vi "TTT_AI.vi"() -> ()   [LabVIEW 2017]
panel:
  in  "Registerkarte":enum32{"Start", "Begr", "spiel", "info"}(tab)
  in  "Eingabe":bool
  in  "Name":string
  out "AnzeigeBegrüß":string
  in  "Registerkarte 2":enum32{"Seite 1"}(tab)
  in  "Panel Farbe":u32(colorbox)
  in  "Panel Farbe 2":u32
  in  "Boolesch":bool
  in  "info1":bool
  in  "spieler1":bool
  out "Ring":u16(ring)
  out "Scoreboard":T1(tab)
  out "Leicht":T2
  out "Mittel":T3
  out "Unmöglich":T3
  out "Mit Fruende":T3
  out "Ausgabe":string
  out "Scoring":bool
  out "O Zug":bool
  in  "X Zug":bool
  in  "BoolArray":bool[][](array[boolean])
  out "Array":i8[][](array[ring])
  in  "Zeile x Spalte":i8=3 min=3 max=3
  in  "stop":bool
  in  "NSpiel":bool
  out "ShowLed":bool
  out "SBeendet":bool
  out "NZueg":i8
  out "O Gewonen":bool
  out "X Gewonen":bool
  in  "Enum":T4(ring)
  in  "zurück":bool
  out "String":string
  out "hidenArray":u8[][](array[numeric])
  # "Geben Sie Ihre Name ein"
  # "Nächte Zug"
  # "Farbe Ändern"
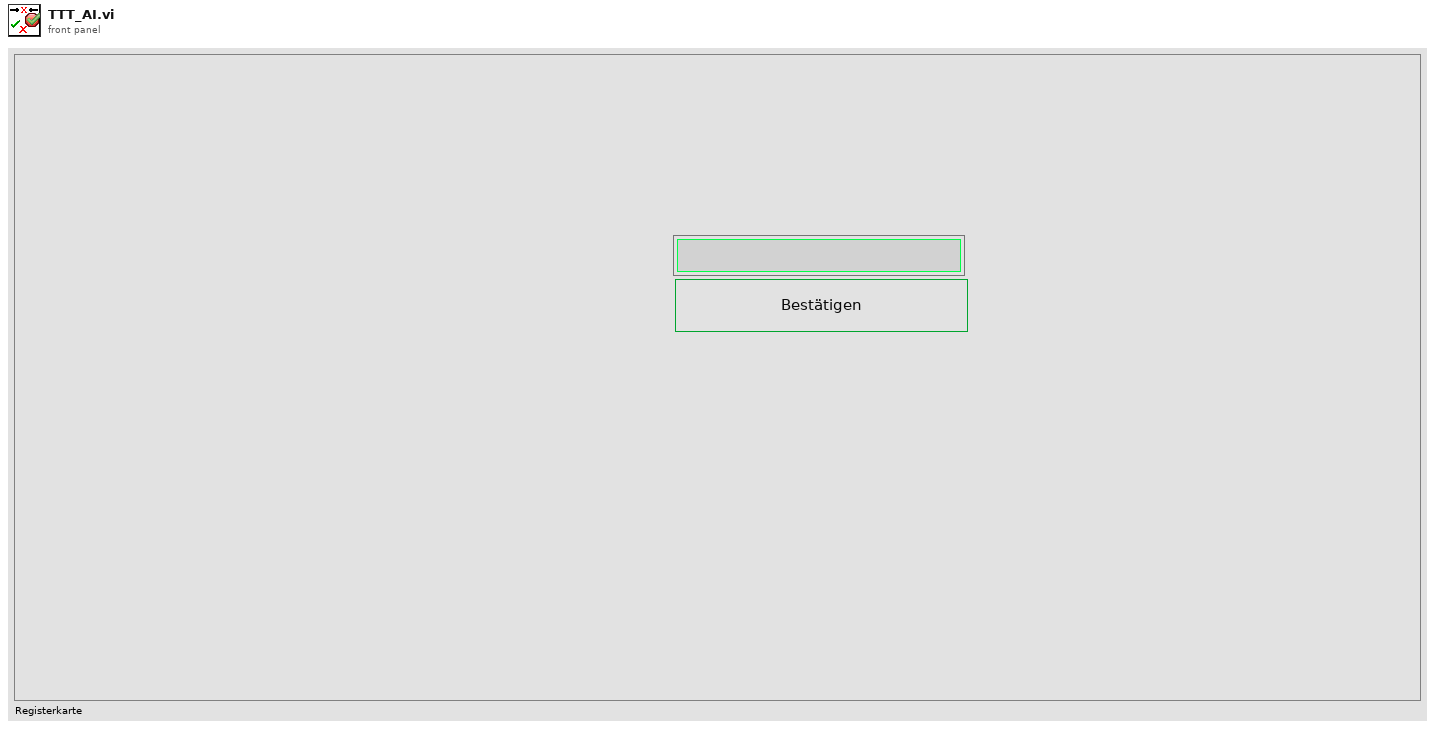
[diagram p1: front panel]
types:
  T1 = enum32{"Seite 1", "Seite 2", "Seite 3", "Seite 4"}
  T2 = cluster{"Spieler":u32, "Gegner":u32, "Unenschieden":u32}
  T3 = cluster{"Spieler":u32, "System":u32, "Unenschieden":u32}
  T4 = enum16{"Leicht", "Mittel", "Unmöglich", "Mit einem Freund Spielen"}
  T5 = enum8{"Enabled", "Disabled", "Disabled and Grayed Out"}
  T6 = cluster{"Spieler":dbl, "Rechner":dbl, "Draw":dbl}
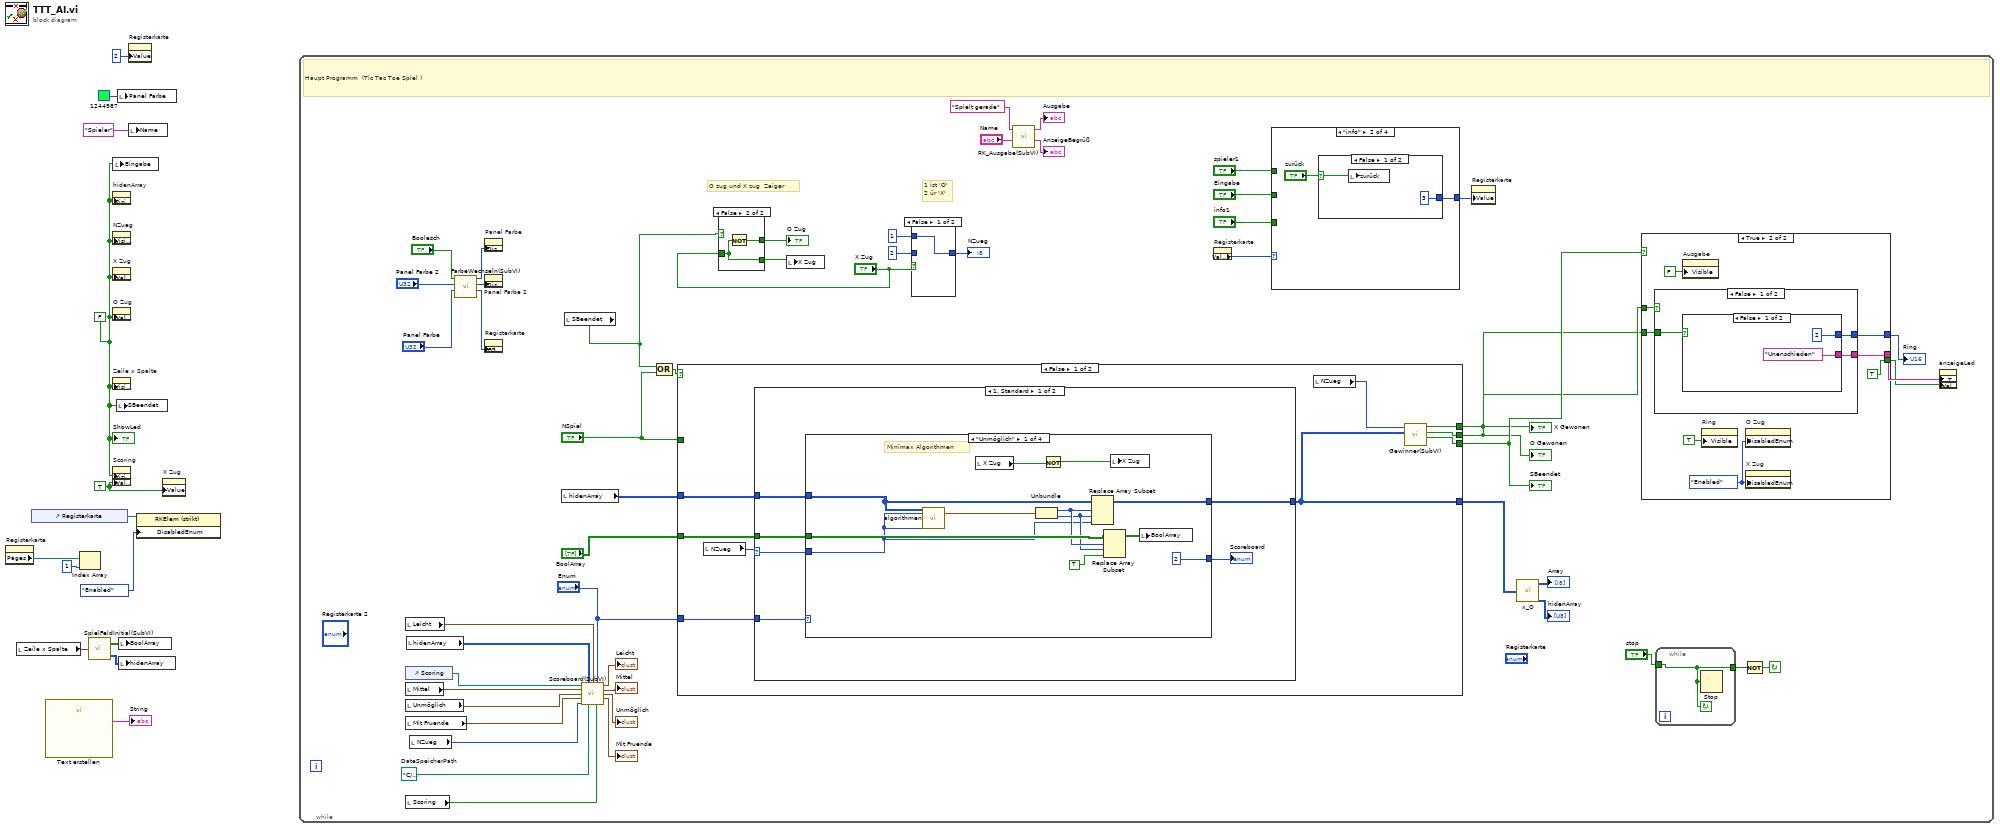
[diagram p0: block diagram]
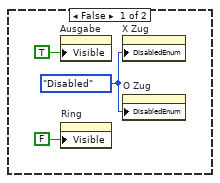
[diagram p3: hidden frame]
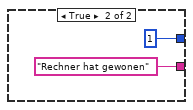
[diagram p4: hidden frame]
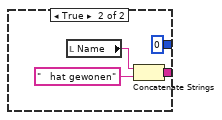
[diagram p5: hidden frame]
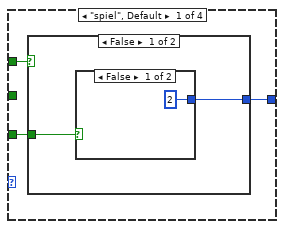
[diagram p6: hidden frame]
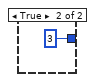
[diagram p7: hidden frame]
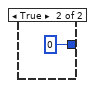
[diagram p8: hidden frame]
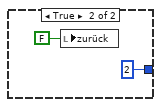
[diagram p9: hidden frame]
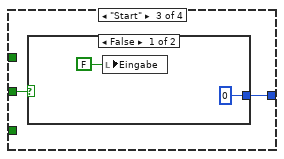
[diagram p10: hidden frame]
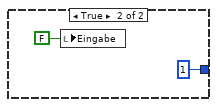
[diagram p11: hidden frame]
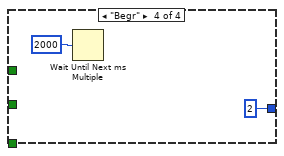
[diagram p12: hidden frame]
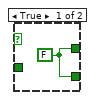
[diagram p13: hidden frame]
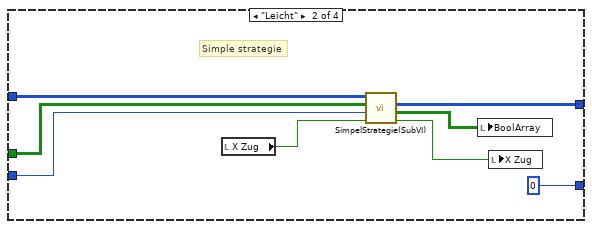
[diagram p14: hidden frame]
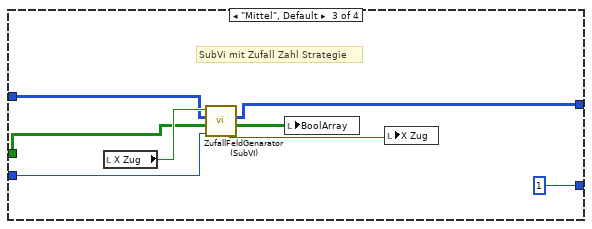
[diagram p15: hidden frame]
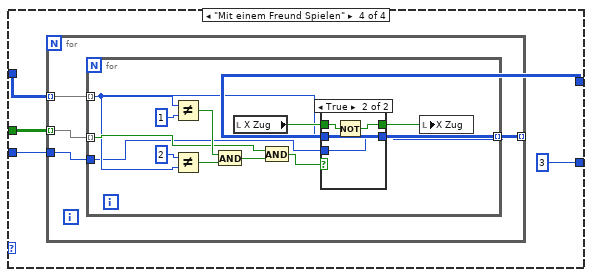
[diagram p16: hidden frame]
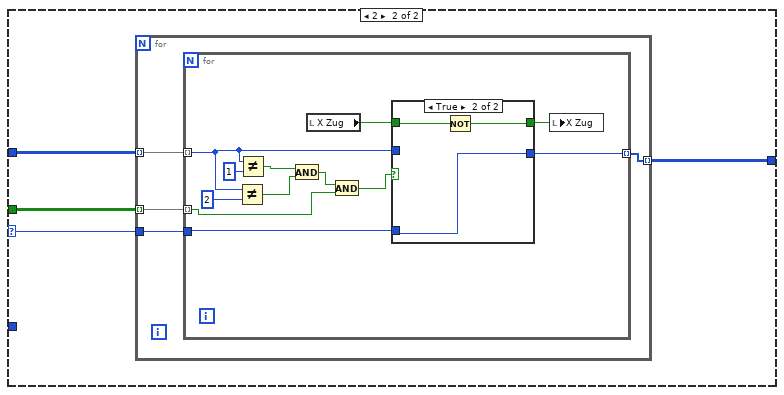
[diagram p18: hidden frame]
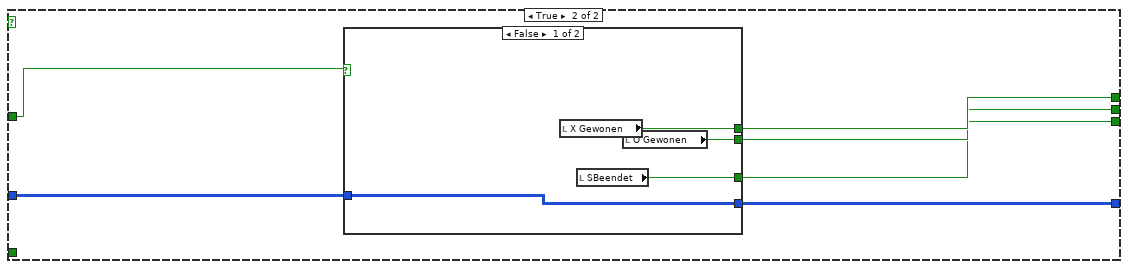
[diagram p20: hidden frame]
diagram:
  w2 = FALSE
  w1 = TRUE
  n1 = property on="Registerkarte" class="RKElem (strikt)"() -> ("Pages"=w6:refnum<vi>[])  [unwired: 2 in, 2 out]
  n2 = local read "Zeile x Spalte"() -> (w13:i8)
  n3 = control-ref of="Registerkarte"() -> (w5:refnum<vi>)
  n4 = call "Text erstellen"() -> ("Result"=→"String":string)  [unwired: 14 in, 1 out]
  n5 = Index Array(array=w6, index=1 ("Index")) -> ()  [unwired: 1 out]
  n6 = call "SpielFeldInitial(SubVI).vi"("SpalteUndZeile"=w13) -> ("TictactoeFelder"=w12:bool[][], "Grafikring"=w11:i8[][])
  n7 = local write "Eingabe"(w2) -> ()
  n8 = property on="hidenArray" class="Arr (strikt)"("Visible"=w2) -> ()  [unwired: 2 in, 2 out]
  n9 = property on="NZueg" class="DigWert (strikt)"("Visible"=w2) -> ()  [unwired: 2 in, 2 out]
  n10 = property on="X Zug" class="Bool. (strikt)"("Value"=w2) -> ()  [unwired: 2 in, 2 out]
  n11 = property on="O Zug" class="Bool. (strikt)"("Value"=w2) -> ()  [unwired: 2 in, 2 out]
  n12 = property on="Zeile x Spalte" class="DigWert (strikt)"("Visible"=w2) -> ()  [unwired: 2 in, 2 out]
  n13 = property on="Scoring" class="Bool. (strikt)"("Visible"=w2, "Value"=w1) -> ()  [unwired: 2 in, 2 out]
  n14 = local write "SBeendet"(w2) -> ()
  n15 = local write "Panel Farbe"(u32 1244987 ("Panel Farbe")) -> ()
  n16 = local write "BoolArray"(w12) -> ()
  n17 = local write "hidenArray"(w11) -> ()
  n18 = property on="Registerkarte" class="RKElem (strikt)"("Value"=2) -> ()  [unwired: 2 in, 2 out]
  n19 = local write "Name"("Spieler") -> ()
  n20 = property class="RKElem (strikt)"(reference=w5, "DisabledEnum"=T5."Enabled" ("Deaktiviert")) -> ()  [unwired: 1 in, 2 out]
  n21 = property on="X Zug" class="Bool. (strikt)"("Value"=w1) -> ()  [unwired: 2 in, 2 out]
  n22 = while {
    stop <- w57 continue-if-true
    w35 = path "C:/Users/MohammadZahirul/Desktop/TicTacToe_Doc/projekt_tictactoe/Ergebnis.txt"  # DateSpeicherPath
    # "O zug und X zug  Zeiger"
    # "1 ist 'O'\n2 ür 'X'"
    # "Haupt Programm  (Tic Tac Toe Spiel )"
    n23 = local read "Leicht"() -> (w55:T2)
    n24 = control-ref of="Scoring"() -> (w43:refnum<vi>)
    n25 = local read "Mittel"() -> (w54:T3)
    n26 = local read "Unmöglich"() -> (w53:T3)
    n27 = local read "Mit Fruende"() -> (w52:T3)
    n28 = local read "Scoring"() -> (w56:bool)
    n29 = local read "hidenArray"() -> (w33:u8[][])
    n30 = local read "NZueg"() -> (w36:i8)
    n31 = call "FarbeWechseln(SubVI).vi"("Panel Farbe"="Panel Farbe", "Panel Farbe 2"="Panel Farbe 2", "Boolesch"="Boolesch") -> ("Panel Farbe 3"=w39:u32, "Deaktiviert 2"=w42:T5, "Deaktiviert"=w40:T5)  [unwired: 6 in]
    n32 = property on="Panel Farbe" class="Farbfeld"("DisabledEnum"=w40) -> ()  [unwired: 2 in, 2 out]
    n33 = property on="Panel Farbe 2" class="DigWert (strikt)"("DisabledEnum"=w42) -> ()  [unwired: 2 in, 2 out]
    n34 = property on="Registerkarte" class="RKElem (strikt)"("FG Color"=w39) -> ()  [unwired: 2 in, 2 out]
    n35 = local read "hidenArray"() -> (w34:u8[][])
    n36 = local read "SBeendet"() -> (w20:bool)
    n37 = call "Scoreboard(SubVI).vi"("Boolean (Eingang)"=w43, "Tic Tac Toe (Eingang)"=w33, "Leicht"=w55, "Enum"="Enum", "Mittel"=w54, "Unmöglich"=w53, "Mit Fruende"=w52, "Next Turn"=w36, "DateSpeicherPath"=w35, "Ergebnis"=w56) -> ("Score 5"=→"Leicht":T6, "Score 6"=→"Mittel":T6, "Score 7"=→"Unmöglich":T6, "Score 8"=→"Mit Fruende":T6)  [unwired: 2 in]
    n38 = Compound Arithmetic op=OR ("Mehrfacharithmetik")(w20, "NSpiel") -> (w65:bool)
    n39 = case shown="False" w65 {
      tunnel: [w122 w215] -> w30
      tunnel: "BoolArray" -> [w124 _]
      tunnel: [w123 w214] -> w29
      tunnel: "NSpiel" -> [_ w211]
      tunnel: w34 -> [w121 w212]
      tunnel: [w119 w213] -> w61
      tunnel: [w120 w210] -> w31
      tunnel: "Enum" -> [w116 _]
      frame False {
        n40 = local read "NZueg"() -> (w117:i8)
        n41 = case shown="1, Standard" w117 {
          selector: w117 -> [w129 w186]
          tunnel: w124 -> [w130 w187]
          tunnel: w121 -> [w128 w188]
          tunnel: [w127 w185] -> w119
          tunnel: w116 -> [w125 _]
          frame 1, Default {
            n42 = case shown="\"Unmöglich\"" w125 {
              tunnel: w130 -> [w140 w146 w156 w163]
              tunnel: w129 -> [w137 w145 w152 w162]
              tunnel: w128 -> [w141 w147 w154 w161]
              tunnel: [w135 w150 w153 w160] -> w127
              tunnel: [2 0 1 3] -> w126
              frame "Unmöglich" {
                # "Minimax Algorithmen"
                n43 = call "algorithmen.vi"("Game"=w141, "Active Turn"=w137, "NextTurn"=w137) -> ("Next Move"=w142:cluster{"Row":i32, "Col":i32})  [unwired: 13 in, 3 out]
                n44 = local read "X Zug"() -> (w133:bool)
                n45 = Unbundle(w142) -> ("Row"=w139:i32, "Col"=w138:i32)
                n46 = Not(x=w133) -> (.not. x?=w132:bool)
                n47 = Replace Array Subset(array=w141, new element=w137, index (row)=w139, index (col)=w138) -> (w135:u8[][])
                n48 = Replace Array Subset(array=w140, new element=TRUE, index (row)=w139, index (col)=w138) -> (w134:bool[][])
                n49 = local write "X Zug"(w132) -> ()
                n50 = local write "BoolArray"(w134) -> ()
              }
              frame "Leicht" {
                # "Simple strategie"
                n51 = local read "X Zug"() -> (w144:bool)
                n52 = call "SimpelStrategie(SubVI).vi"("toggle"=w144, "NextTurn"=w145, "BoolArray"=w146, "Array"=w147) -> ("toggle 2"=w148:bool, "Array 3"=w149:bool[][], "Array 2"=w150:u8[][])  [unwired: 1 in]
                n53 = local write "BoolArray"(w149) -> ()
                n54 = local write "X Zug"(w148) -> ()
              }
              frame "Mittel", Default {
                # "SubVi mit Zufall Zahl Strategie"
                n55 = local read "X Zug"() -> (w157:bool)
                n56 = call "ZufallFeldGenarator (SubVI).vi"("Numerisch"=w152, "BoolArray (Eingang)"=w156, "Tic Tac Toe (Eingang)"=w154, "Toggle turn (Eingang)"=w157) -> ("BoolArray (Ausgang)"=w155:bool[][], "Tic Tac Toe (Ausgang)"=w153:u8[][], "Toggle turn (Ausgang)"=w158:bool)  [unwired: 1 in]
                n57 = local write "BoolArray"(w155) -> ()
                n58 = local write "X Zug"(w158) -> ()
              }
              frame "Mit einem Freund Spielen" {
                n59 = for {
                  tunnel: w163 -> [w167] mode=indexing
                  tunnel: w162 -> [w166]
                  tunnel: w161 -> [w165] mode=indexing
                  tunnel: [w164] -> w160 mode=indexing
                  n60 = for {
                    tunnel: w167 -> [w176] mode=indexing
                    tunnel: w166 -> [w168]
                    tunnel: w165 -> [w170] mode=indexing
                    tunnel: [w169] -> w164 mode=indexing
                    n61 = Not Equal?(x=w170, y=1) -> (x != y?=w179:bool)
                    n62 = Not Equal?(x=2, y=w170) -> (x != y?=w178:bool)
                    n63 = And(x=w179, y=w178) -> (x .and. y?=w177:bool)
                    n64 = local read "X Zug"() -> (w173:bool)
                    n65 = And(x=w176, y=w177) -> (x .and. y?=w175:bool)
                    n66 = case shown="True" w175 {
                      tunnel: [w181 w184] -> w174
                      tunnel: w173 -> [w181 w183]
                      tunnel: [w180 w182] -> w169
                      tunnel: w170 -> [w180 _]
                      tunnel: w168 -> [_ w182]
                      frame False {
                      }
                      frame True {
                        n67 = Not(x=w183) -> (.not. x?=w184:bool)
                      }
                    }
                    n68 = local write "X Zug"(w174) -> ()
                  }
                }
              }
            }
            "Scoreboard" <- w126
          }
          frame 2 {
            n69 = for {
              tunnel: w188 -> [w192] mode=indexing
              tunnel: w187 -> [w191] mode=indexing
              tunnel: w186 -> [w190]
              tunnel: [w189] -> w185 mode=indexing
              n70 = for {
                tunnel: w192 -> [w195] mode=indexing
                tunnel: w191 -> [w199] mode=indexing
                tunnel: w190 -> [w197]
                tunnel: [w196] -> w189 mode=indexing
                n71 = Not Equal?(x=w195, y=u8 2) -> (x != y?=w201:bool)
                n72 = Not Equal?(x=w195, y=u8 1) -> (x != y?=w202:bool)
                n73 = And(x=w202, y=w201) -> (x .and. y?=w200:bool)
                n74 = local read "X Zug"() -> (w194:bool)
                n75 = And(x=w200, y=w199) -> (x .and. y?=w198:bool)
                n76 = case shown="True" w198 {
                  tunnel: w197 -> [_ w209]
                  tunnel: [w206 w209] -> w196
                  tunnel: w195 -> [w206 _]
                  tunnel: w194 -> [w205 w207]
                  tunnel: [w205 w208] -> w193
                  frame False {
                  }
                  frame True {
                    n77 = Not(x=w207) -> (.not. x?=w208:bool)
                  }
                }
                n78 = local write "X Zug"(w193) -> ()
              }
            }
          }
        }
        n79 = local read "NZueg"() -> (w118:i8)
        n80 = call "Gewinner(SubVI).vi"("Array"=w119, "Next Turn"=w118) -> ("Game over"=w120:bool, "Win 2"=w123:bool, "Win"=w122:bool)  [unwired: 7 in]
      }
      frame True {
        n81 = case shown="False" w211 {
          tunnel: [w218 w226] -> w215
          tunnel: [w219 w226] -> w214
          tunnel: [w217 w223] -> w213
          tunnel: w212 -> [w217 _]
          tunnel: [w216 w226] -> w210
          frame False {
            n82 = local read "X Gewonen"() -> (w218:bool)
            n83 = local read "SBeendet"() -> (w216:bool)
            n84 = local read "O Gewonen"() -> (w219:bool)
          }
          frame True {
            w226 = FALSE
            n85 = property on="X Zug" class="Bool. (strikt)"("Value"=TRUE) -> ()  [unwired: 2 in, 2 out]
            n86 = call "SpielFeldInitial(SubVI).vi"("SpalteUndZeile"="Zeile x Spalte") -> ("TictactoeFelder"=w224:bool[][], "Grafikring"=w223:i8[][])
            n87 = local write "NZueg"(i8 2 ("Next Turn")) -> ()
            n88 = local write "BoolArray"(w224) -> ()
            "Scoring" <- TRUE
          }
        }
      }
    }
    "X Gewonen" <- w30
    "O Gewonen" <- w29
    "SBeendet" <- w31
    n89 = case shown="False" w20 {
      tunnel: [w112 w114] -> w22
      tunnel: [w112 w113] -> w23
      tunnel: "X Zug" -> [_ w114]
      frame True {
        w112 = FALSE
      }
      frame False {
        n90 = Not(x=w114) -> (.not. x?=w113:bool)
      }
    }
    "O Zug" <- w23
    n91 = local write "X Zug"(w22) -> ()
    n92 = case shown="False" "X Zug" {
      tunnel: [w66 w67] -> w26
      tunnel: 1 -> [w66 _]
      tunnel: 2 -> [_ w67]
      frame False {
      }
      frame True {
      }
    }
    "NZueg" <- w26
    n93 = call "RK_Ausgabe(SubVI).vi"("Name"="Name", "werS"="Spielt gerade") -> ("AnzeigeBegrüß"=→"AnzeigeBegrüß":string, "AnzeigeOben"=→"Ausgabe":string)  [unwired: 8 in]
    n94 = property on="Registerkarte" class="RKElem (strikt)"() -> ("Value"=w60:enum32{"Start", "Begr", "spiel", "info"})  [unwired: 2 in, 2 out]
    n95 = case shown="\"info\"" w60 {
      tunnel: [w92 w98 w105 2] -> w17
      tunnel: "Eingabe" -> [_ _ w104 _]
      tunnel: "spieler1" -> [w91 _ _ _]
      tunnel: "info1" -> [w90 _ _ _]
      frame "spiel", Default {
        n96 = case shown="False" w91 {
          tunnel: [w94 0] -> w92
          tunnel: w90 -> [w93 _]
          frame False {
            n97 = case shown="False" w93 {
              tunnel: [2 3] -> w94
              frame False {
              }
              frame True {
              }
            }
          }
          frame True {
          }
        }
      }
      frame "info" {
        n98 = case shown="False" "zurück" {
          selector: "zurück" -> [w100 _]
          tunnel: [3 2] -> w98
          frame False {
            n99 = local write "zurück"(w100) -> ()
          }
          frame True {
            n100 = local write "zurück"(FALSE) -> ()
          }
        }
      }
      frame "Start" {
        n101 = case shown="False" w104 {
          tunnel: [0 1] -> w105
          frame False {
            n102 = local write "Eingabe"(FALSE) -> ()
          }
          frame True {
            n103 = local write "Eingabe"(FALSE) -> ()
          }
        }
      }
      frame "Begr" {
        n104 = Wait Until Next ms Multiple(millisecond multiple=u32 2000 ("ms")) -> ()  [unwired: 1 out]
      }
    }
    n105 = property on="Registerkarte" class="RKElem (strikt)"("Value"=w17) -> ()  [unwired: 2 in, 2 out]
    n106 = call "x_O.vi"("Tic Tac Toe"=w61) -> ("GrafikRing"=→"Array":i32[][], "Game"=→"hidenArray":i32[][])  [unwired: 8 in]
    n107 = case shown="True" w31 {
      tunnel: w30 -> [_ w78]
      tunnel: w29 -> [_ w77]
      tunnel: [_ w76] -> w28
      tunnel: [_ w74] -> w27
      tunnel: [_ TRUE] -> w18
      frame False {
        w69 = T5."Disabled" ("Deaktiviert")
        n108 = property on="Ausgabe" class="Str"("Visible"=TRUE ("Sichtbar")) -> ()  [unwired: 2 in, 2 out]
        n109 = property on="Ring" class="Ring (strikt)"("Visible"=FALSE) -> ()  [unwired: 2 in, 2 out]
        n110 = property on="X Zug" class="Bool. (strikt)"("DisabledEnum"=w69) -> ()  [unwired: 2 in, 2 out]
        n111 = property on="O Zug" class="Bool. (strikt)"("DisabledEnum"=w69) -> ()  [unwired: 2 in, 2 out]
      }
      frame True {
        w73 = T5."Enabled" ("Deaktiviert")
        n112 = case shown="False" w78 {
          tunnel: w77 -> [w81 _]
          tunnel: [w80 0] -> w76
          tunnel: [w79 w88] -> w74
          frame False {
            n113 = case shown="False" w81 {
              tunnel: [2 1] -> w80
              tunnel: ["Unenschieden" "Rechner hat gewonen"] -> w79
              frame False {
              }
              frame True {
              }
            }
          }
          frame True {
            n114 = local read "Name"() -> (w87:string)
            n115 = Concatenate Strings(w87, "   hat gewonen" ("String")) -> (w88:string)
          }
        }
        n116 = property on="Ausgabe" class="Str"("Visible"=FALSE ("Sichtbar")) -> ()  [unwired: 2 in, 2 out]
        n117 = property on="Ring" class="Ring (strikt)"("Visible"=TRUE) -> ()  [unwired: 2 in, 2 out]
        n118 = property on="O Zug" class="Bool. (strikt)"("DisabledEnum"=w73) -> ()  [unwired: 2 in, 2 out]
        n119 = property on="X Zug" class="Bool. (strikt)"("DisabledEnum"=w73) -> ()  [unwired: 2 in, 2 out]
      }
    }
    "Ring" <- w28
    n120 = while {
      tunnel: "stop" -> [w115]
      tunnel: [w115] -> w44
      stop <- w115 continue-if-true
      n121 = Stop(stop? (T)=w115) -> ()
    }
    n122 = Not(x=w44) -> (.not. x?=w57:bool)
    n123 = property on="anzeigeLed" class="Bool. (strikt)"("BoolText.Text"=w27, "Value"=w18) -> ()  [unwired: 2 in, 2 out]
  }
  "ShowLed" <- w2
